vi "ChangeField.vi"(0 "Starting Field (T)":dbl format="%.2f", 2 "Desired Field (T)":dbl format="%.3f", 3 "Magnet System":enum16{"Resistive", "Hybrid"}(ring), 5 "error in (no error)":errorcluster) -> (4 "Status":cluster{bool, bool, "Ramp Status":u16, bool}, 6 "Tesla":dbl(knob) caption="Current Field (T)" min=0.02 max=0.03072874735534784 scale=0.20023601171997402..0.3 scale format="%#_4g", 8 "error out":errorcluster)   [LabVIEW 2020]
uses:
  Globals and TypeDefs/Type Definitions.llb/3 way Status.ctl
  Globals and TypeDefs/Error Categories.ctt
  <vilib>/Utility/error.llb/DialogType.ctl
  Globals and TypeDefs/gStatus.vi
  Globals and TypeDefs/gHField.vi
panel:
  out "ChangeField Status":T1(ring)
  in  "Tolerance (T)":dbl=0.003 min=0.0001 max=1.0 step=0.0001 format="%.3f"
  in  "stop":bool
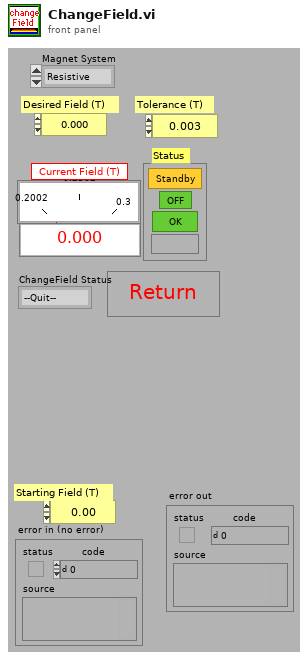
[diagram p1: front panel]
types:
  T1 = enum16{"--Quit--", "Read Initial Status", "Set New Field", "Check Field Value"}
  T2 = typedef "3 way Status.ctl" = u8
  T3 = enum16{"--Quit--", "Read-Status", "Read-Cell", "Read-Field[T]", "Read-Setpoint[T]"}
  T4 = enum8{"Initialization Error", "Command Error", "Parameter Error", "Overflow Error", "Time-out Error", "Misc Error", "User cancel"}
  T5 = typedef "Error Categories.ctt" = enum8{"General", "CCD-256x1024", "CCD-1340x400", "InGaAs PDA", "McPherson 2075", "Magnetic Field", "Temperature Control", "Other"}
  T6 = cluster{"PS on/off":bool, "PS fault?":bool, "Ramp Status":u16, "PS Control?":bool}
  T7 = typedef "DialogType.ctl" = u16
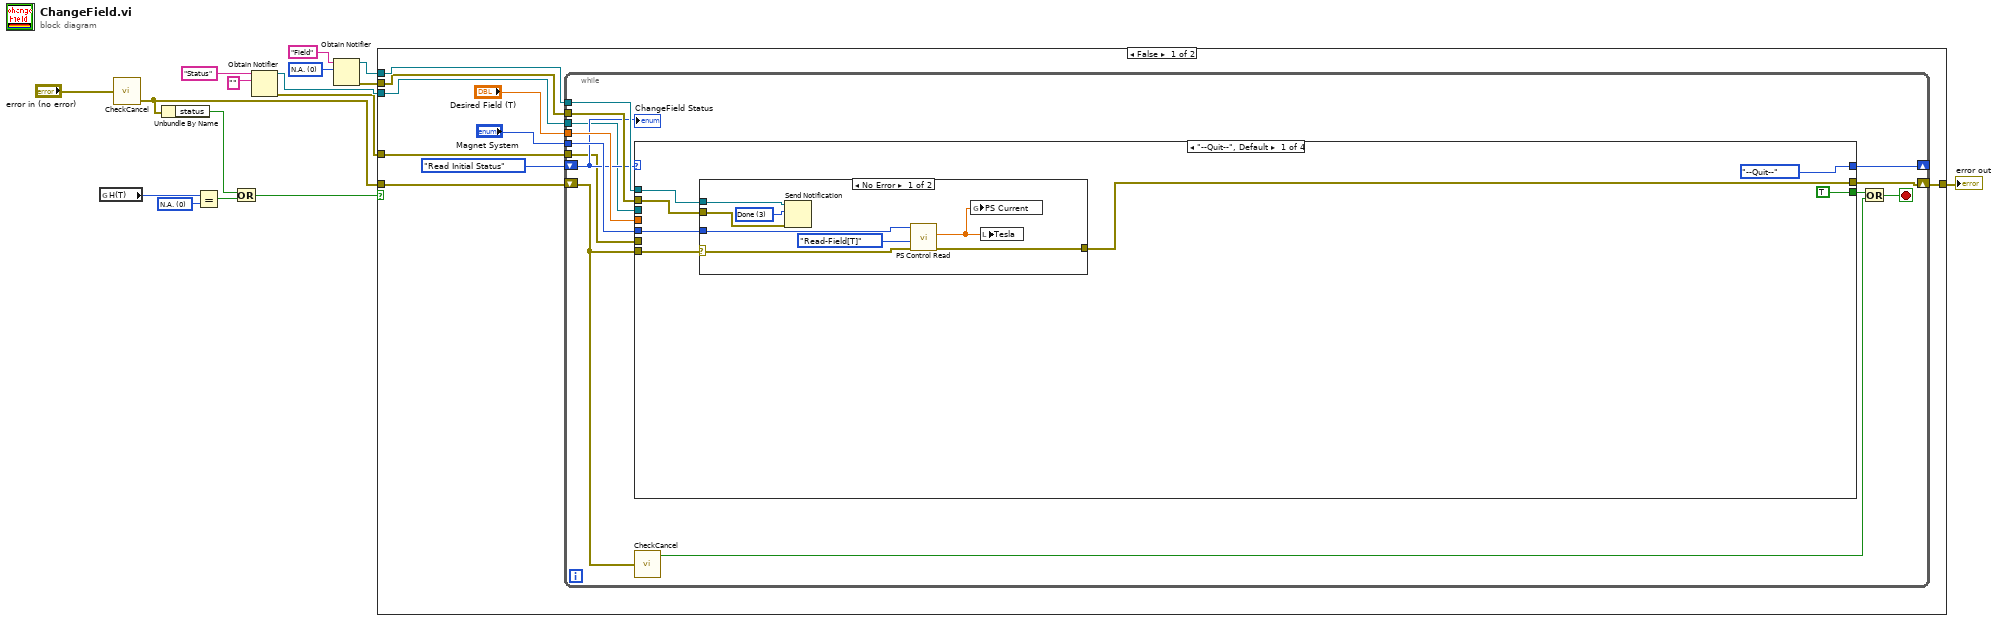
[diagram p0: block diagram]
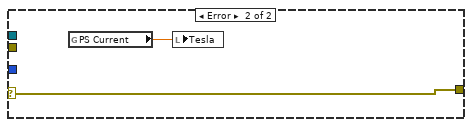
[diagram p2: hidden frame]
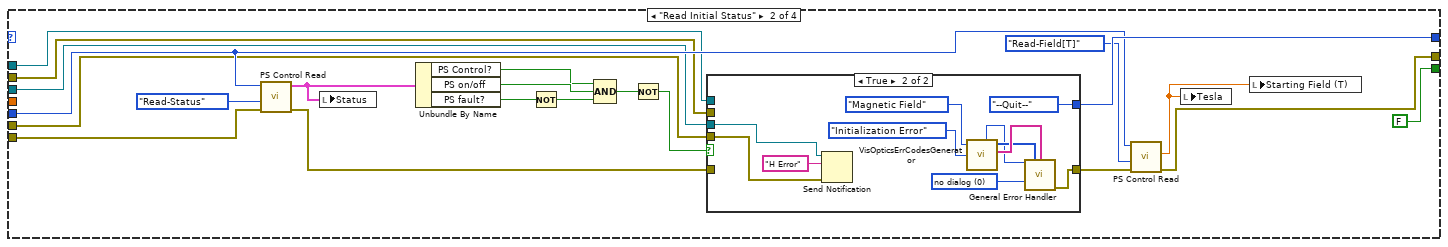
[diagram p3: hidden frame]
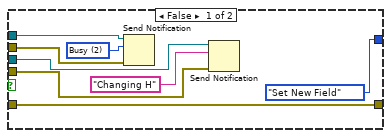
[diagram p4: hidden frame]
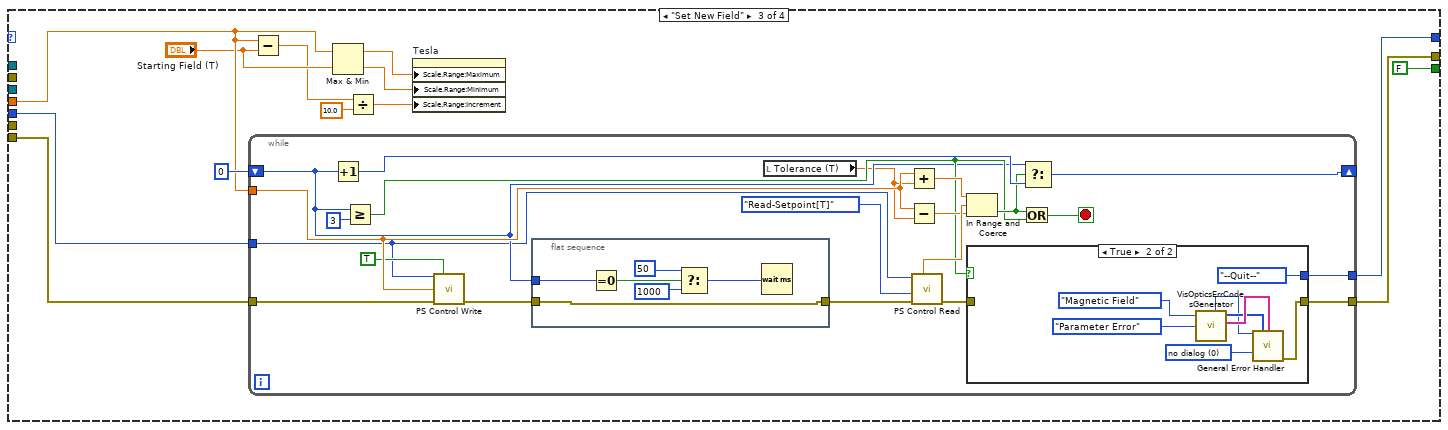
[diagram p5: hidden frame]
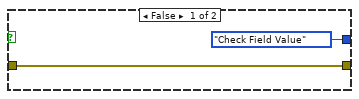
[diagram p6: hidden frame]
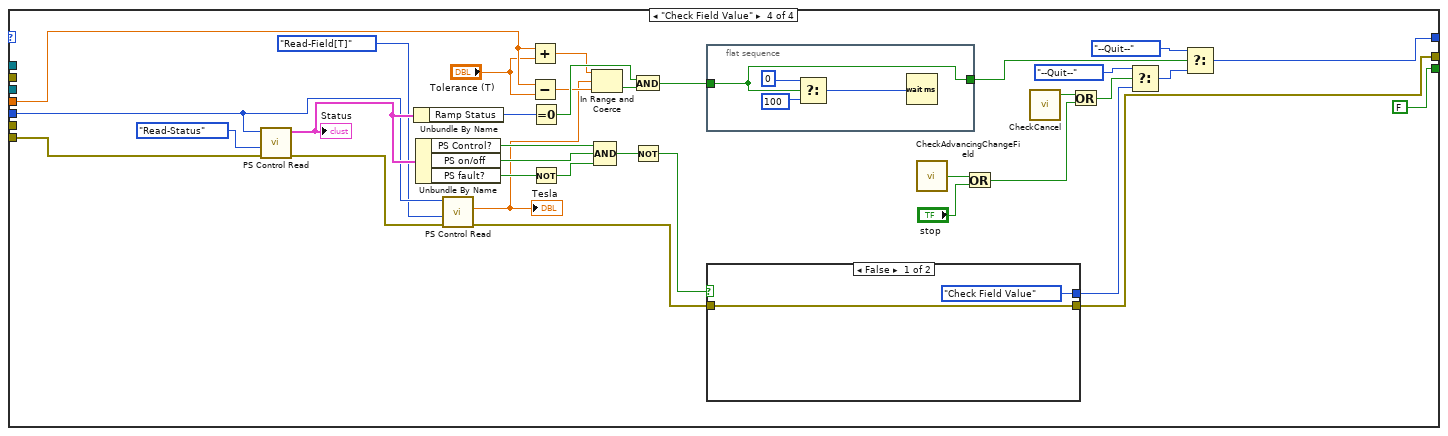
[diagram p7: hidden frame]
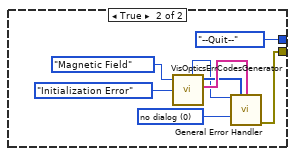
[diagram p8: hidden frame]
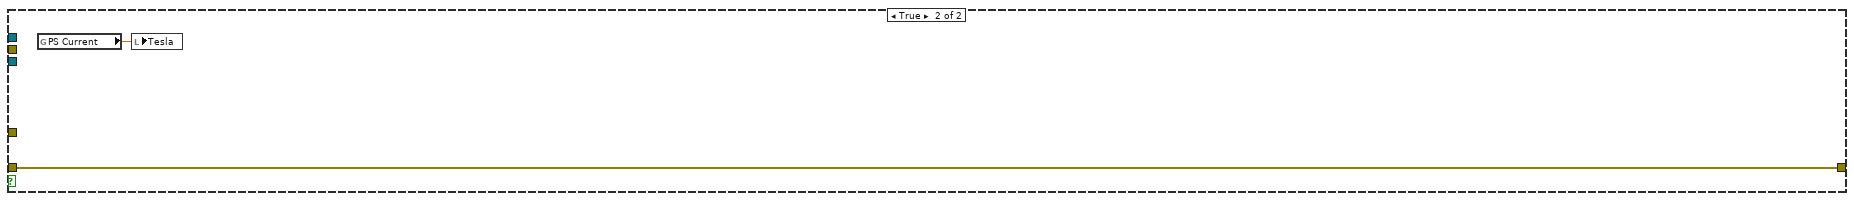
[diagram p9: hidden frame]
diagram:
  w9 = T2 0 items=["N.A.", "OK", "Busy", "Done"] ("Saving")
  w16 = T2 0 items=["N.A.", "OK", "Busy", "Done"] ("y")
  n1 = global read "gStatus.vi" "H(T)"() -> (w15:T2)
  n2 = call "CheckCancel.vi"("error in (no error)"="error in (no error)") -> ("error out"=w2:errorcluster)  [unwired: 1 in, 1 out]
  n3 = Unbundle By Name(w2) -> ("status"=w13:bool)
  n4 = Equal?(x=w15, y=w16) -> (x = y?=w11:bool)
  n5 = Or(x=w13, y=w11) -> (x .or. y?=w14:bool)
  n6 = Obtain Notifier(name (unnamed)="Status", notification data type="" ("Status")) -> (notifier out=w4:refnum<notifier>, error out=w3:errorcluster)  [unwired: 2 in, 1 out]
  n7 = Obtain Notifier(name (unnamed)="Field", notification data type=w9) -> (notifier out=w8:refnum<notifier>, error out=w7:errorcluster)  [unwired: 2 in, 1 out]
  n8 = case shown="False" w14 {
    tunnel: w2 -> [w23 w196]
    tunnel: [w22 w196] -> w12
    tunnel: w8 -> [w21 _]
    tunnel: w7 -> [w20 _]
    tunnel: w4 -> [w18 _]
    tunnel: w3 -> [w17 _]
    frame False {
      n9 = while {
        shift-right: [w37] -> w22
        shift-left: w23 -> [w32]
        tunnel: "Magnet System" -> [w38]
        tunnel: "Desired Field (T)" -> [w36]
        tunnel: w21 -> [w31]
        tunnel: w20 -> [w30]
        shift-right: [w29] -> _
        shift-left: T1."Read Initial Status" ("ChangeField Status") -> [w28]
        tunnel: w18 -> [w27]
        tunnel: w17 -> [w26]
        stop <- w35 stop-if-true
        n10 = case shown="\"--Quit--\", Default" w28 {
          tunnel: w32 -> [w44 w71 w107 w176]
          tunnel: w38 -> [w43 w62 w108 w156]
          tunnel: [w42 w63 w105 w168] -> w37
          tunnel: w36 -> [_ _ w100 w160]
          tunnel: [T1."--Quit--" ("ChangeField Status") w67 w104 w169] -> w29
          tunnel: [TRUE FALSE FALSE FALSE] -> w34
          tunnel: w31 -> [w41 w59 _ _]
          tunnel: w30 -> [w40 w58 _ _]
          tunnel: w27 -> [_ w57 _ _]
          tunnel: w26 -> [_ w56 _ _]
          frame "--Quit--", Default {
            n11 = case shown="No Error" w44 {
              selector: w44 -> [w51 w55]
              tunnel: w43 -> [w53 _]
              tunnel: [w50 w55] -> w42
              tunnel: w41 -> [w49 _]
              tunnel: w40 -> [w48 _]
              frame No Error {
                w47 = T2 3 items=["N.A.", "OK", "Busy", "Done"] ("H(T)")
                n12 = Send Notification(notification=w47, notifier=w49, error in (no error)=w48) -> ()  [unwired: 2 out]
                n13 = call "PS Control Read.vi"("error in"=w51, "Read State"=T3."Read-Field[T]", "Magnet System"=w53) -> ("error out"=w50:errorcluster, "Current Field"=w46:dbl)  [unwired: 1 in, 3 out]
                n14 = global write "gHField.vi" "PS Current"(w46) -> ()
                n15 = local write "Tesla"(w46) -> ()
              }
              frame Error {
                n16 = global read "gHField.vi" "PS Current"() -> (w54:dbl)
                n17 = local write "Tesla"(w54) -> ()
              }
            }
          }
          frame "Read Initial Status" {
            n18 = call "PS Control Read.vi"("error in"=w71, "Read State"=T3."Read-Status", "Magnet System"=w62) -> ("error out"=w70:errorcluster, "Status"=w74:T6)  [unwired: 1 in, 3 out]
            n19 = local write "Status"(w74) -> ()
            n20 = Unbundle By Name(w74) -> ("PS Control?"=w75:bool, "PS on/off"=w76:bool, "PS fault?"=w72:bool)
            n21 = Not(x=w72) -> (.not. x?=w73:bool)
            n22 = Compound Arithmetic op=AND(w75, w76, w73) -> (w68:bool)
            n23 = Not(x=w68) -> (.not. x?=w69:bool)
            n24 = case shown="True" w69 {
              tunnel: [w84 w90] -> w64
              tunnel: w70 -> [w84 _]
              tunnel: [T1."Set New Field" ("ChangeField Status") T1."--Quit--" ("ChangeField Status")] -> w67
              tunnel: w59 -> [w83 _]
              tunnel: w58 -> [w82 _]
              tunnel: w57 -> [w79 w86]
              tunnel: w56 -> [w78 w85]
              frame False {
                w81 = T2 2 items=["N.A.", "OK", "Busy", "Done"] ("H(T)")
                n25 = Send Notification(notification=w81, notifier=w83, error in (no error)=w82) -> ()  [unwired: 2 out]
                n26 = Send Notification(notification="Changing H", notifier=w79, error in (no error)=w78) -> ()  [unwired: 2 out]
              }
              frame True {
                w95 = T7 0 items=["no dialog", "OK message", "continue or stop message", "OK message + warnings", "continue/stop + warnings"] ("type of dialog (OK msg:1)")
                n27 = Send Notification(notification="H Error", notifier=w86, error in (no error)=w85) -> ()  [unwired: 2 out]
                n28 = call "VisOpticsErrCodesGenerator.vi"("NHMFL Visible Optics Error Type"=T4."Initialization Error", "NHMFL Visible Optics Error Categories"=Error_Categories.ctt."Magnetic Field") -> ("user-defined descriptions"=w94:string[], "User-defined Error Code"=w89:i32, "user-defined codes"=w93:i32[])  [unwired: 1 in, 3 out]
                n29 = call <vilib>:"General Error Handler.vi"("[error code] (0)"=w89, "[user-defined codes]"=w93, "[user-defined descriptions]"=w94, "type of dialog (OK msg:1)"=w95) -> ("error out"=w90:errorcluster)  [unwired: 7 in, 4 out]
              }
            }
            n30 = call "PS Control Read.vi"("error in"=w64, "Read State"=T3."Read-Field[T]", "Magnet System"=w62) -> ("error out"=w63:errorcluster, "Current Field"=w60:dbl)  [unwired: 1 in, 3 out]
            n31 = local write "Tesla"(w60) -> ()
            n32 = local write "Starting Field (T)"(w60) -> ()
          }
          frame "Set New Field" {
            n33 = while {
              tunnel: w108 -> [w110]
              tunnel: w100 -> [w123]
              tunnel: w107 -> [w129]
              shift-right: [w121] -> _
              shift-left: u8 0 ("Desired Field (T)") -> [w113]
              tunnel: [w115] -> w105
              tunnel: [w114] -> w104
              stop <- w118 stop-if-true
              n34 = Increment(x=w113) -> (x+1=w122:u8)
              n35 = Greater Or Equal?(x=w113, y=u8 3) -> (x >= y?=w117:bool)
              n36 = call "PS Control Write.vi"("Magnet System"=w110, "Ramp"=TRUE, "Setpoint"=w123, "error in (no error)"=w129) -> ("error out"=w128:errorcluster)  [unwired: 10 in, 1 out]
              n37 = flat-sequence {
                tunnel: [w145] -> w127
                tunnel: w128 -> [w145]
                tunnel: w113 -> [w144]
                frame #0 {
                  n38 = Equal To 0?(x=w144) -> (x = 0?=w143:bool)
                  n39 = Select(t=u32 50 ("milliseconds to wait"), s=w143, f=u32 1000) -> (s? t:f=w141:u32)
                  n40 = Wait (ms)(milliseconds to wait=w141) -> ()  [unwired: 1 out]
                }
              }
              n41 = local read "Tolerance (T)"() -> (w109:dbl)
              n42 = Add(x=w123, y=w109) -> (x+y=w125:dbl)
              n43 = Subtract(x=w123, y=w109) -> (x-y=w124:dbl)
              n44 = call "PS Control Read.vi"("error in"=w127, "Read State"=T3."Read-Setpoint[T]", "Magnet System"=w110) -> ("error out"=w116:errorcluster, "Current Setpoint (T)"=w126:dbl)  [unwired: 1 in, 3 out]
              n45 = In Range and Coerce(upper limit=w125, x=w126, lower limit=w124) -> (In Range?=w119:bool)  [unwired: 1 out]
              n46 = case shown="True" w117 {
                tunnel: [w131 w134] -> w115
                tunnel: w116 -> [w131 _]
                tunnel: [T1."Check Field Value" ("ChangeField Status") T1."--Quit--" ("ChangeField Status")] -> w114
                frame False {
                }
                frame True {
                  w139 = T7 0 items=["no dialog", "OK message", "continue or stop message", "OK message + warnings", "continue/stop + warnings"] ("type of dialog (OK msg:1)")
                  n47 = call "VisOpticsErrCodesGenerator.vi"("NHMFL Visible Optics Error Type"=T4."Parameter Error", "NHMFL Visible Optics Error Categories"=Error_Categories.ctt."Magnetic Field") -> ("user-defined descriptions"=w138:string[], "User-defined Error Code"=w133:i32, "user-defined codes"=w137:i32[])  [unwired: 1 in, 3 out]
                  n48 = call <vilib>:"General Error Handler.vi"("[error code] (0)"=w133, "[user-defined codes]"=w137, "[user-defined descriptions]"=w138, "type of dialog (OK msg:1)"=w139) -> ("error out"=w134:errorcluster)  [unwired: 7 in, 4 out]
                }
              }
              n49 = Or(x=w119, y=w117) -> (x .or. y?=w118:bool)
              n50 = Select(t=w113, s=w119, f=w122) -> (s? t:f=w121:u8)
            }
            n51 = Subtract(x=w100, y="Starting Field (T)") -> (x-y=w98:dbl)
            n52 = Max & Min(x=w100, y="Starting Field (T)") -> (max(x,y)=w102:dbl, min(x,y)=w101:dbl)
            n53 = Divide(x=w98, y=10.0) -> (x/y=w96:dbl)
            n54 = property on="Tesla" class="Knob (strict)"("Scale.Range:Maximum"=w102, "Scale.Range:Minimum"=w101, "Scale.Range:Increment"=w96) -> ()  [unwired: 2 in, 2 out]
          }
          frame "Check Field Value" {
            n55 = call "PS Control Read.vi"("error in"=w176, "Read State"=T3."Read-Status", "Magnet System"=w156) -> ("error out"=w157:errorcluster, "Status"=w175:T6)  [unwired: 1 in, 3 out]
            "Status" <- w175
            n56 = Unbundle By Name(w175) -> ("Ramp Status"=w173:u16)
            n57 = Unbundle By Name(w175) -> ("PS Control?"=w179:bool, "PS on/off"=w180:bool, "PS fault?"=w177:bool)
            n58 = call "PS Control Read.vi"("error in"=w157, "Read State"=T3."Read-Field[T]", "Magnet System"=w156) -> ("error out"=w153:errorcluster, "Current Field"=w154:dbl)  [unwired: 1 in, 3 out]
            "Tesla" <- w154
            n59 = Add(x=w160, y="Tolerance (T)") -> (x+y=w164:dbl)
            n60 = Subtract(x=w160, y="Tolerance (T)") -> (x-y=w163:dbl)
            n61 = Equal To 0?(x=w173) -> (x = 0?=w172:bool)
            n62 = Not(x=w177) -> (.not. x?=w178:bool)
            n63 = In Range and Coerce(upper limit=w164, x=w154, lower limit=w163) -> (In Range?=w171:bool)  [unwired: 1 out]
            n64 = Compound Arithmetic op=AND(w179, w180, w178) -> (w162:bool)
            n65 = And(x=w172, y=w171) -> (x .and. y?=w166:bool)
            n66 = Not(x=w162) -> (.not. x?=w161:bool)
            n67 = flat-sequence {
              tunnel: [w181] -> w165
              tunnel: w166 -> [w181]
              frame #0 {
                n68 = Select(t=u32 0 ("milliseconds to wait"), s=w181, f=u32 100) -> (s? t:f=w183:u32)
                n69 = Wait (ms)(milliseconds to wait=w183) -> ()  [unwired: 1 out]
              }
            }
            n70 = case shown="False" w161 {
              tunnel: [w186 w189] -> w168
              tunnel: w153 -> [w186 _]
              tunnel: [T1."Check Field Value" ("ChangeField Status") T1."--Quit--" ("ChangeField Status")] -> w174
              frame False {
              }
              frame True {
                w194 = T7 0 items=["no dialog", "OK message", "continue or stop message", "OK message + warnings", "continue/stop + warnings"] ("type of dialog (OK msg:1)")
                n71 = call "VisOpticsErrCodesGenerator.vi"("NHMFL Visible Optics Error Type"=T4."Initialization Error", "NHMFL Visible Optics Error Categories"=Error_Categories.ctt."Magnetic Field") -> ("user-defined descriptions"=w193:string[], "User-defined Error Code"=w188:i32, "user-defined codes"=w192:i32[])  [unwired: 1 in, 3 out]
                n72 = call <vilib>:"General Error Handler.vi"("[error code] (0)"=w188, "[user-defined codes]"=w192, "[user-defined descriptions]"=w193, "type of dialog (OK msg:1)"=w194) -> ("error out"=w189:errorcluster)  [unwired: 7 in, 4 out]
              }
            }
            n73 = call "CheckAdvancingChangeField.vi"() -> ("Advancing"=w149:bool)  [unwired: 1 in]
            n74 = Or(x=w149, y="stop") -> (x .or. y?=w147:bool)
            n75 = call "CheckCancel.vi"() -> ("Cancelled"=w148:bool)  [unwired: 2 in, 1 out]
            n76 = Or(x=w148, y=w147) -> (x .or. y?=w146:bool)
            n77 = Select(t=T1."--Quit--" ("ChangeField Status"), s=w146, f=w174) -> (s? t:f=w170:T1)
            n78 = Select(t=T1."--Quit--" ("ChangeField Status"), s=w165, f=w170) -> (s? t:f=w169:T1)
          }
        }
        n79 = call "CheckCancel.vi"("error in (no error)"=w32) -> ("Cancelled"=w33:bool)  [unwired: 1 in, 1 out]
        n80 = Or(x=w34, y=w33) -> (x .or. y?=w35:bool)
        "ChangeField Status" <- w28
      }
    }
    frame True {
      n81 = global read "gHField.vi" "PS Current"() -> (w195:dbl)
      n82 = local write "Tesla"(w195) -> ()
    }
  }
  "error out" <- w12
